vi "1B_EditGenCalData.vi"(0 "Gen Cal Data In":string) -> (4 "Gen Cal Data Out":string)   [LabVIEW 2010]
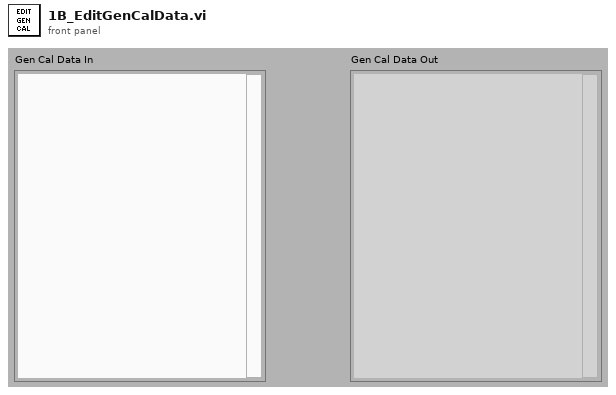
[diagram p1: front panel]
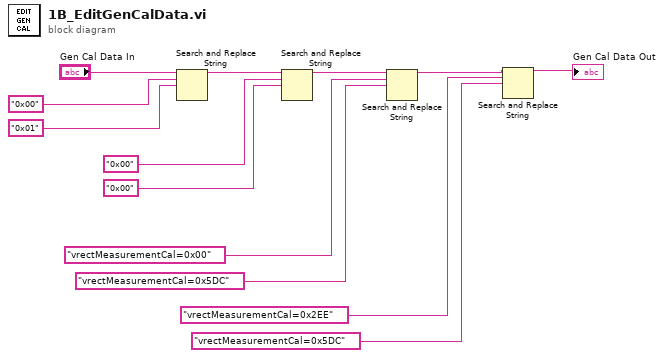
[diagram p0: block diagram]
diagram:
  n1 = Search and Replace String(input string="Gen Cal Data In", search string="0x00", replace string="0x01") -> (result string=w12:string)  [unwired: 5 in, 3 out]
  n2 = Search and Replace String(input string=w12, search string="0x00", replace string="0x00") -> (result string=w11:string)  [unwired: 5 in, 3 out]
  n3 = Search and Replace String(input string=w11, search string="vrectMeasurementCal=0x00", replace string="vrectMeasurementCal=0x5DC") -> (result string=w2:string)  [unwired: 5 in, 3 out]
  n4 = Search and Replace String(input string=w2, search string="vrectMeasurementCal=0x2EE", replace string="vrectMeasurementCal=0x5DC") -> (result string=→"Gen Cal Data Out":string)  [unwired: 5 in, 3 out]
